vi "StateMachineTest.vi"() -> ()   [LabVIEW 2019]
uses:
  StateMachineTest_State.vi
panel:
  in  "Stop":bool
  in  "Start":bool
  out "LED3":bool
  out "LED2":bool
  out "LED1":bool
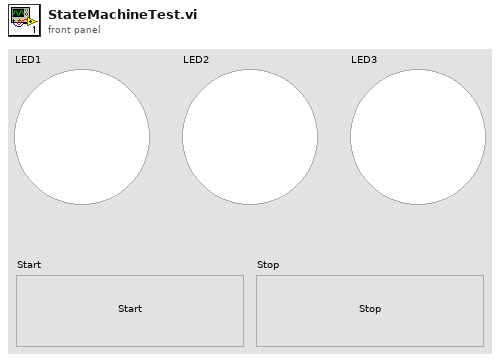
[diagram p1: front panel]
types:
  T1 = typedef "StateMachineTest_State.vi" = enum16{"Idle", "LED1", "LED2", "LED3"}
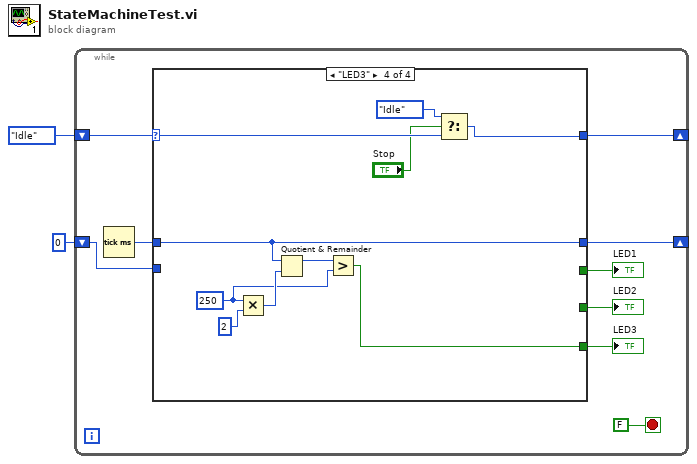
[diagram p0: block diagram]
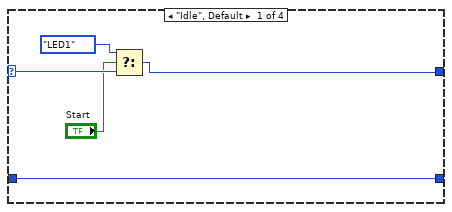
[diagram p2: hidden frame]
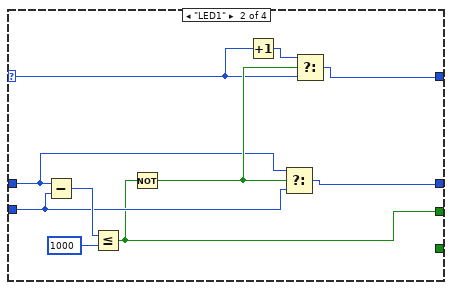
[diagram p3: hidden frame]
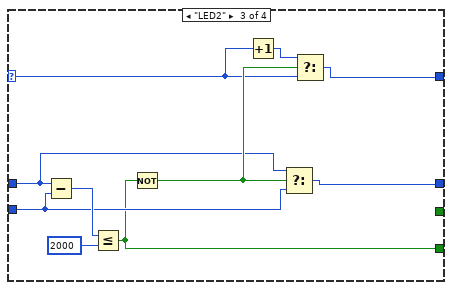
[diagram p4: hidden frame]
diagram:
  n1 = while {
    shift-right: [w10] -> _
    shift-left: StateMachineTest_State.vi."Idle" -> [w11]
    shift-right: [w8] -> _
    shift-left: u32 0 ("millisecond timer value") -> [w7]
    stop <- FALSE stop-if-true
    n2 = Tick Count (ms)() -> (millisecond timer value=w9:u32)
    n3 = case shown="\"LED3\"" w11 {
      selector: w11 -> [w16 w19 w29 w45]
      tunnel: [w14 w20 w30 w46] -> w10
      tunnel: w9 -> [w13 w21 w31 w44]
      tunnel: [w13 w22 w32 w44] -> w8
      tunnel: w7 -> [_ w23 w33 _]
      tunnel: [_ _ w27 _] -> w5
      tunnel: [_ w17 _ _] -> w4
      tunnel: [_ _ _ w38] -> w3
      frame "Idle", Default {
        n4 = Select(t=StateMachineTest_State.vi."LED1", s="Start", f=w16) -> (s? t:f=w14:T1)
      }
      frame "LED1" {
        n5 = Subtract(x=w21, y=w23) -> (x-y=w25:u32)
        n6 = Less Or Equal?(x=w25, y=u32 1000) -> (x <= y?=w17:bool)
        n7 = Not(x=w17) -> (.not. x?=w26:bool)
        n8 = Increment(x=w19) -> (x+1=w18:T1)
        n9 = Select(t=w21, s=w26, f=w23) -> (s? t:f=w22:u32)
        n10 = Select(t=w18, s=w26, f=w19) -> (s? t:f=w20:T1)
      }
      frame "LED2" {
        n11 = Subtract(x=w31, y=w33) -> (x-y=w35:u32)
        n12 = Less Or Equal?(x=w35, y=u32 2000) -> (x <= y?=w27:bool)
        n13 = Not(x=w27) -> (.not. x?=w36:bool)
        n14 = Increment(x=w29) -> (x+1=w28:T1)
        n15 = Select(t=w31, s=w36, f=w33) -> (s? t:f=w32:u32)
        n16 = Select(t=w28, s=w36, f=w29) -> (s? t:f=w30:T1)
      }
      frame "LED3" {
        w40 = u32 250 ("y")
        n17 = Multiply(x=w40, y=u32 2) -> (x*y=w42:u32)
        n18 = Quotient & Remainder(x=w44, y=w42) -> (x-y*floor(x/y)=w41:u32)  [unwired: 1 out]
        n19 = Greater?(x=w41, y=w40) -> (0:w38:bool)
        n20 = Select(t=StateMachineTest_State.vi."Idle", s="Stop", f=w45) -> (s? t:f=w46:T1)
      }
    }
    "LED2" <- w5
    "LED1" <- w4
    "LED3" <- w3
  }
